vi "Jeffress_model_v001.vi"() -> ()   [LabVIEW 2019]
panel:
  out "Get Start Time (s) 2":dbl caption="Get Start Time (s)"
  out "Get Start Time (s)":dbl
  out "Delay RL":dbl
  out "Delay LR":dbl
  in  "stop":bool
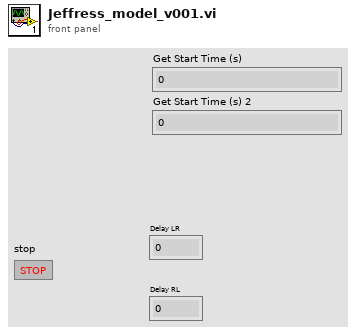
[diagram p1: front panel]
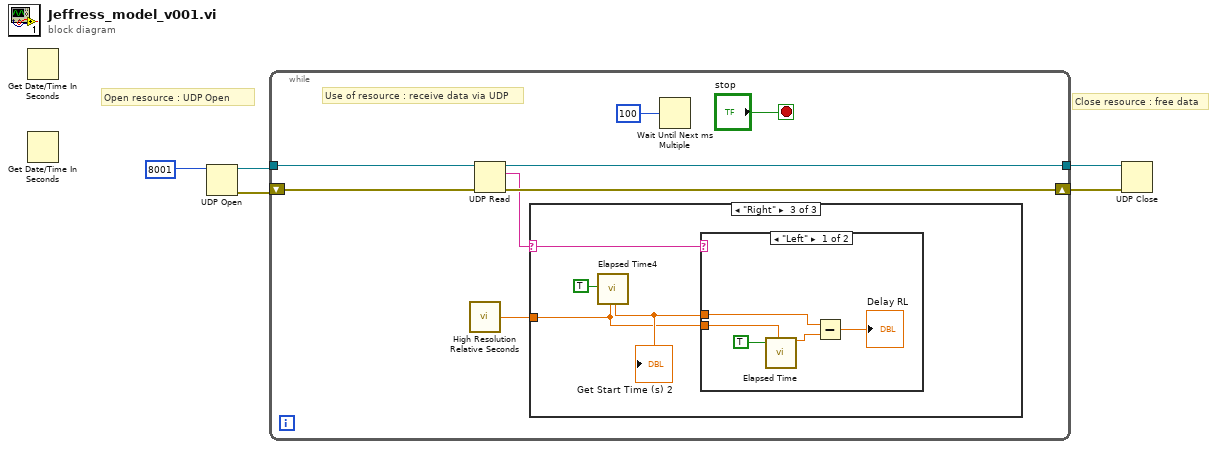
[diagram p0: block diagram]
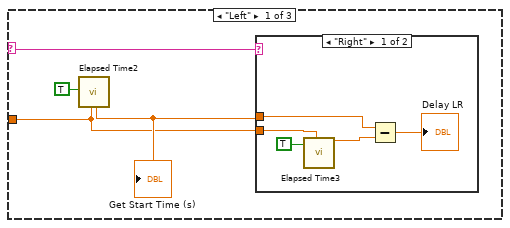
[diagram p2: hidden frame]
diagram:
  # "Close resource : free data"
  # "Open resource : UDP Open"
  n1 = Get Date/Time In Seconds() -> ()  [unwired: 1 out]
  n2 = Get Date/Time In Seconds() -> ()  [unwired: 1 out]
  n3 = UDP Open(11:u16 8001) -> (port=w3:refnum<k16>, 0:w5:errorcluster)  [unwired: 4 in, 1 out]
  n4 = while {
    tunnel: w3 -> [w9]
    tunnel: [w8] -> w2
    shift-right: [w11] -> w4
    shift-left: w5 -> [w10]
    stop <- "stop" stop-if-true
    # "Use of resource : receive data via UDP"
    n5 = call <vilib>:"High Resolution Relative Seconds.vi"() -> ("relative seconds"=w6:dbl)
    n6 = UDP Read(connection ID=w9, 8:w10) -> (data out=w7:string, error out=w11:errorcluster, 3:w8:refnum<k16>)  [unwired: 2 in, 2 out]
    n7 = case shown="\"Right\"" w7 {
      selector: w7 -> [w17 _ w25]
      tunnel: w6 -> [w15 _ w24]
      frame "Left" {
        n8 = call "Elapsed Time2"("Reset"=TRUE, "Set Start Time (s)"=w15) -> ("Get Start Time (s)"=w16:dbl)  [unwired: 10 in, 7 out]
        "Get Start Time (s)" <- w16
        n9 = case shown="\"Right\"" w17 {
          tunnel: w16 -> [w20 _]
          tunnel: w15 -> [w22 _]
          frame "Right" {
            n10 = call "Elapsed Time3"("Reset"=TRUE, "Set Start Time (s)"=w22) -> ("Present (s)"=w19:dbl)  [unwired: 10 in, 7 out]
            n11 = Subtract(x=w20, y=w19) -> (x-y=→"Delay LR":dbl)
          }
          frame "Left", Default {
          }
        }
      }
      frame Default {
      }
      frame "Right" {
        n12 = call "Elapsed Time4"("Reset"=TRUE, "Set Start Time (s)"=w24) -> ("Get Start Time (s)"=w26:dbl)  [unwired: 10 in, 7 out]
        "Get Start Time (s) 2" <- w26
        n13 = case shown="\"Left\"" w25 {
          tunnel: w26 -> [w30 _]
          tunnel: w24 -> [w28 _]
          frame "Left" {
            n14 = call "Elapsed Time"("Reset"=TRUE, "Set Start Time (s)"=w28) -> ("Present (s)"=w29:dbl)  [unwired: 10 in, 7 out]
            n15 = Subtract(x=w30, y=w29) -> (x-y=→"Delay RL":dbl)
          }
          frame "RIght", Default {
          }
        }
      }
    }
    n16 = Wait Until Next ms Multiple(millisecond multiple=u32 100) -> ()  [unwired: 1 out]
  }
  n17 = UDP Close(connection ID=w2, 8:w4) -> ()  [unwired: 2 out]
